vi "Thermal Chamber Controller_DQMH_Action Update Ramp Rate-test_harness.vi"(11 "test case ID":string) -> (3 "result":bool)   [LabVIEW 2018]
doc: "The harness VI is executed for every test case. InstaCoverage passes the test case ID before the execution of the test case in the <b>test case ID</b> input and reads the <b>result</b> output after the execution. If the result is TRUE and no error happens during the execution, then the test case is evaluated as PASSED. If the result is false and no error happens during the execution, then the test case is evaluated as FAILED. Otherwise the test case is evaluated as ERROR.\n\nThe result of the test suite will be PASSED (FAILED) if all (at least one) test cases are PASSED (FAILED). If at least one test case in the test suite has the ERROR result, then the test suite will have ERROR result.\n\n<b>Note: </b>Don't change the connector pane of this VI.\n\nSee the Help Document for more information. (<b>Help</b> > <b>IncQuery Labs</b> > <b>InstaCoverage</b> > <b>InstaCoverage Help...</b>)"
uses:
  Libraries/Thermal Chamber Controller_DQMH/Thermal Chamber Controller_DQMH.lvlib
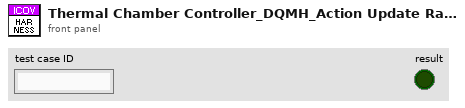
[diagram p1: front panel]
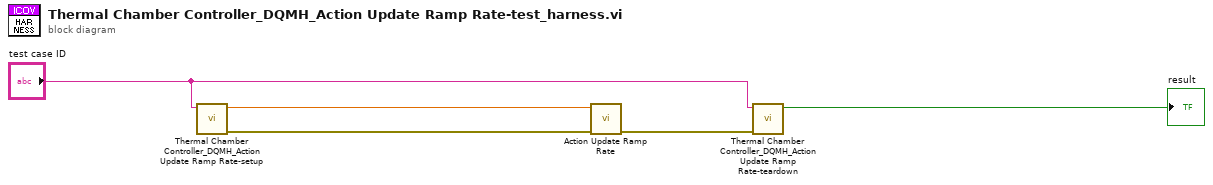
[diagram p0: block diagram]
diagram:
  n1 = call "Thermal Chamber Controller_DQMH_Action Update Ramp Rate-setup.vi"("test case ID"="test case ID") -> ("error in"=w3:errorcluster, "Temperature Ramp Rate"=w4:dbl)  [unwired: 9 in]
  n2 = call "Action Update Ramp Rate.vi"("error in (no error)"=w3, "Temperature Ramp Rate"=w4) -> ("error out"=w2:errorcluster)  [unwired: 9 in]
  n3 = call "Thermal Chamber Controller_DQMH_Action Update Ramp Rate-teardown.vi"("error out"=w2, "test case ID"="test case ID") -> ("result"=→"result":bool)  [unwired: 9 in]
